vi "Set Test Settings.vi"(10 "Test Settings":T1, 11 "Manual Mode Command in":refnum<class "Manual Mode Command.lvclass">) -> (3 "Manual Mode Command out":refnum<class "Manual Mode Command.lvclass">)   [LabVIEW 2016, in "Manual Mode Command.lvclass"]
uses:
  Manual Mode Command.lvclass
  Typedefs/TestSettings.ctl
  Manual Mode Command.lvclass/Manual Mode Command.ctl
  Typedefs/HPMT_Typedefs.lvlib
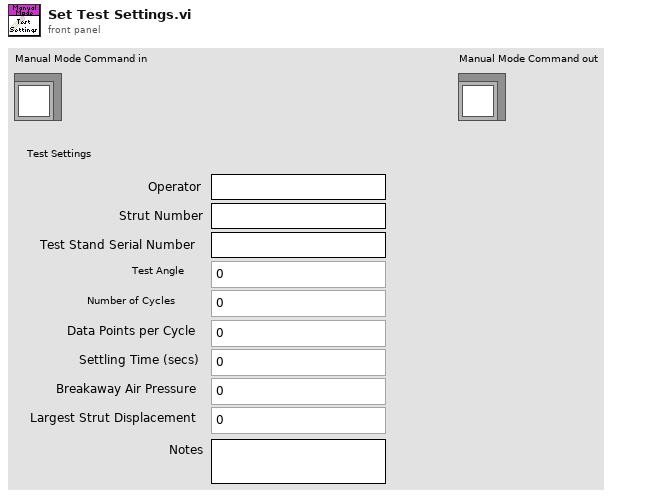
[diagram p1: front panel]
types:
  T1 = typedef "HPMT_Typedefs.lvlib/TestSettings.ctl" = cluster{"Operator":string, "Strut Number":string, "Test Stand Serial Number":string, "Notes":string, "Test Angle":u16, "Number of Cycles":u16, "Data Points per Cycle":u16, "Settling Time (secs)":u16, "Breakaway Air Pressure":u16, "Largest Strut Displacement":dbl}
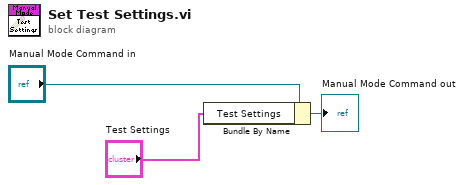
[diagram p0: block diagram]
diagram:
  n1 = Bundle By Name(cluster="Manual Mode Command in", "Test Settings"="Test Settings") -> (→"Manual Mode Command out":refnum<class "Manual Mode Command.lvclass">)
